vi "Get User List.vi"(11 "error in (no error)":errorcluster) -> (8 "Names":string[](array[string]), 10 "SU?":bool[](array[boolean]), 15 "error out":errorcluster)   [LabVIEW 2011]
doc: "Get list of users and User status from Users.cnf"
uses:
  <vilib>/Utility/libraryn.llb/Check if File or Folder Exists.vi
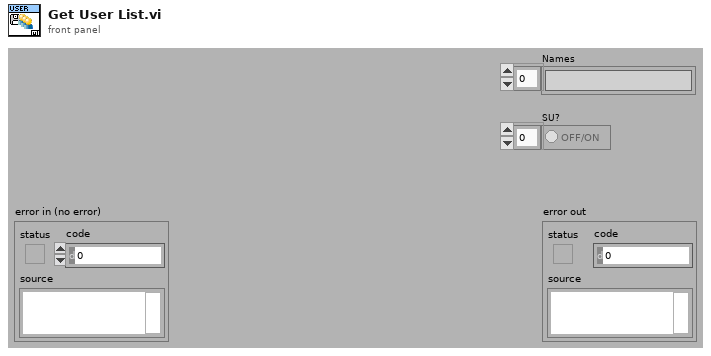
[diagram p1: front panel]
types:
  T1 = enum16{"open", "replace", "create", "open or create", "replace or create", "replace or create with confirmation"}
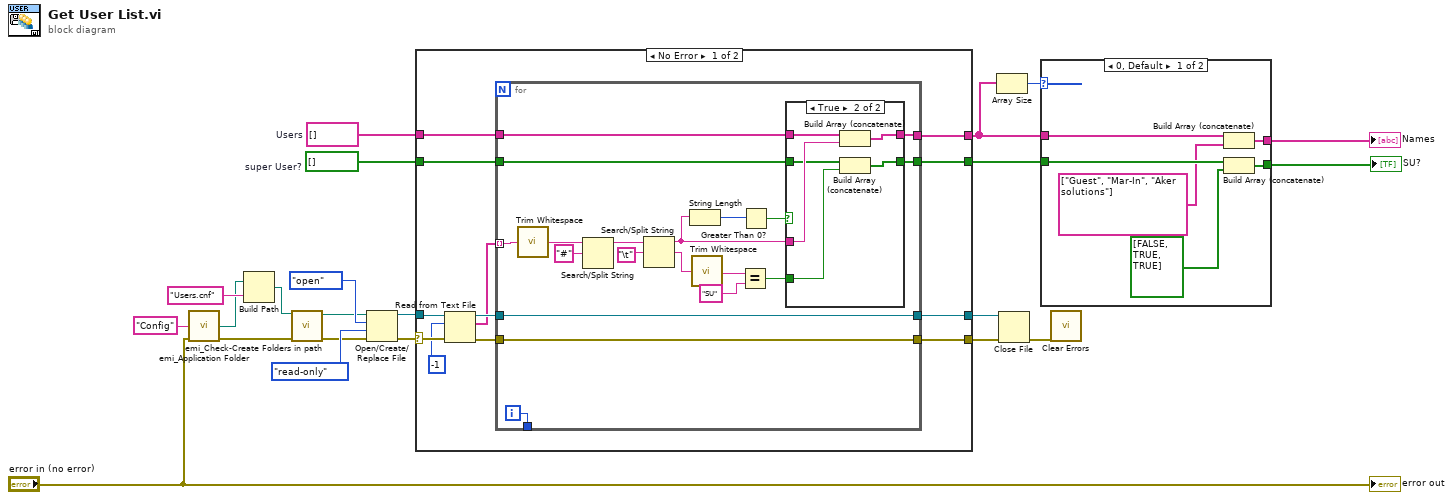
[diagram p0: block diagram]
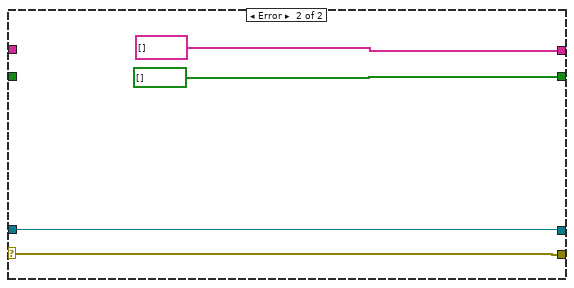
[diagram p4: hidden frame]
diagram:
  w13 = bool[] []  # super User?
  w14 = string[] []  # Users
  n1 = call "emi_Application Folder.vi"("Sub Dir name"="Config" ("Name"), "error in (no error)"="error in (no error)") -> ("Dir"=w6:path, "error out"=w3:errorcluster)  [unwired: 12 in]
  n2 = Build Path(base path=w6, name or relative path="Users.cnf") -> (appended path=w4:path)
  n3 = call "emi_Check-Create Folders in path.vi"("Path including file"=w4, "error in (no error)"=w3) -> ("Path out"=w1:path, "error out"=w2:errorcluster)  [unwired: 11 in, 1 out]
  n4 = Open/Create/Replace File(file path (use dialog)=w1, error in=w2, operation (0:open)=T1."open", access (0:read/write)=enum16{"read/write", "read-only", "write-only"}."read-only") -> (refnum out=w18:refnum<file>, error out=w19:errorcluster)  [unwired: 2 in, 1 out]
  n5 = case shown="No Error" w19 {
    selector: w19 -> [w34 w62]
    tunnel: w18 -> [w33 w63]
    tunnel: [w30 w63] -> w16
    tunnel: [w29 w62] -> w17
    tunnel: w14 -> [w26 _]
    tunnel: w13 -> [w25 _]
    tunnel: [w24 string[] [] ("Users")] -> w11
    tunnel: [w23 bool[] [] ("super User?")] -> w10
    frame No Error {
      n6 = Read from Text File(file (use dialog)=w33, count=-1, error in=w34) -> (refnum out=w31:refnum<file>, text=w28:string[], error out=w32:errorcluster)  [unwired: 1 in, 1 out]
      n7 = for {
        tunnel: w32 -> [w52]
        tunnel: w31 -> [w53]
        tunnel: [w53] -> w30
        tunnel: [w52] -> w29
        tunnel: w28 -> [w51] mode=indexing
        tunnel: w26 -> [w40]
        tunnel: w25 -> [w39]
        tunnel: [w38] -> w24
        tunnel: [w37] -> w23
        tunnel: [w35] -> _
        i -> [w35]
        n8 = call <vilib>:"Trim Whitespace.vi"("string"=w51) -> ("trimmed string"=w50:string)  [unwired: 1 in]
        n9 = Search/Split String(string=w50, search string/char (-)="#") -> (substring before match=w47:string)  [unwired: 1 in, 2 out]
        n10 = Search/Split String(string=w47, search string/char (-)="\t") -> (substring before match=w41:string, match + rest of string=w46:string)  [unwired: 1 in, 1 out]
        n11 = String Length(string=w41) -> (length=w43:i32)
        n12 = call <vilib>:"Trim Whitespace.vi"("string"=w46) -> ("trimmed string"=w45:string)  [unwired: 1 in]
        n13 = Equal?(x=w45, y="SU") -> (x = y?=w36:bool)
        n14 = Greater Than 0?(x=w43) -> (x > 0?=w42:bool)
        n15 = case shown="True" w42 {
          tunnel: w41 -> [_ w59]
          tunnel: w40 -> [w55 w61]
          tunnel: w39 -> [w54 w58]
          tunnel: [w55 w60] -> w38
          tunnel: [w54 w56] -> w37
          tunnel: w36 -> [_ w57]
          frame False {
          }
          frame True {
            n16 = Build Array (concatenate)(w61, w59) -> (w60:string[])
            n17 = Build Array (concatenate)(w58, w57) -> (w56:bool[])
          }
        }
      }
    }
    frame Error {
    }
  }
  n18 = Array Size(array=w11) -> (size(s)=w12:i32)
  n19 = Close File(refnum=w16, error in=w17) -> (error out=w15:errorcluster)  [unwired: 1 out]
  n20 = case shown="0, Default" w12 {
    tunnel: w11 -> [w71 w73]
    tunnel: w10 -> [w70 w72]
    tunnel: [w67 w73] -> w9
    tunnel: [w66 w72] -> w8
    frame 0, Default {
      n21 = Build Array (concatenate)(w71, string[] ["Guest", "Mar-In", "Aker solutions"] ("Users")) -> (w67:string[])
      n22 = Build Array (concatenate)(w70, bool[] [FALSE, TRUE, TRUE] ("super User?")) -> (w66:bool[])
    }
    frame 2.. {
    }
  }
  "Names" <- w9
  "SU?" <- w8
  n23 = call <vilib>:"Clear Errors.vi"("error in (no error)"=w15) -> ()  [unwired: 6 in, 1 out]
  "error out" <- "error in (no error)"
